vi "Calibrate_Open_All_Freqs-OLD.vi"() -> ()   [LabVIEW 2020]
uses:
  HP 4275A Address constant.vi
panel:
  out "error out":errorcluster
  in  "Cal_Delay_Step":u16
  in  "error in":errorcluster
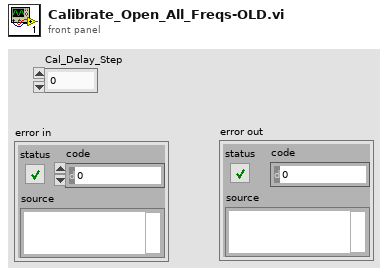
[diagram p1: front panel]
types:
  T1 = typedef "Control 1.ctl" = string
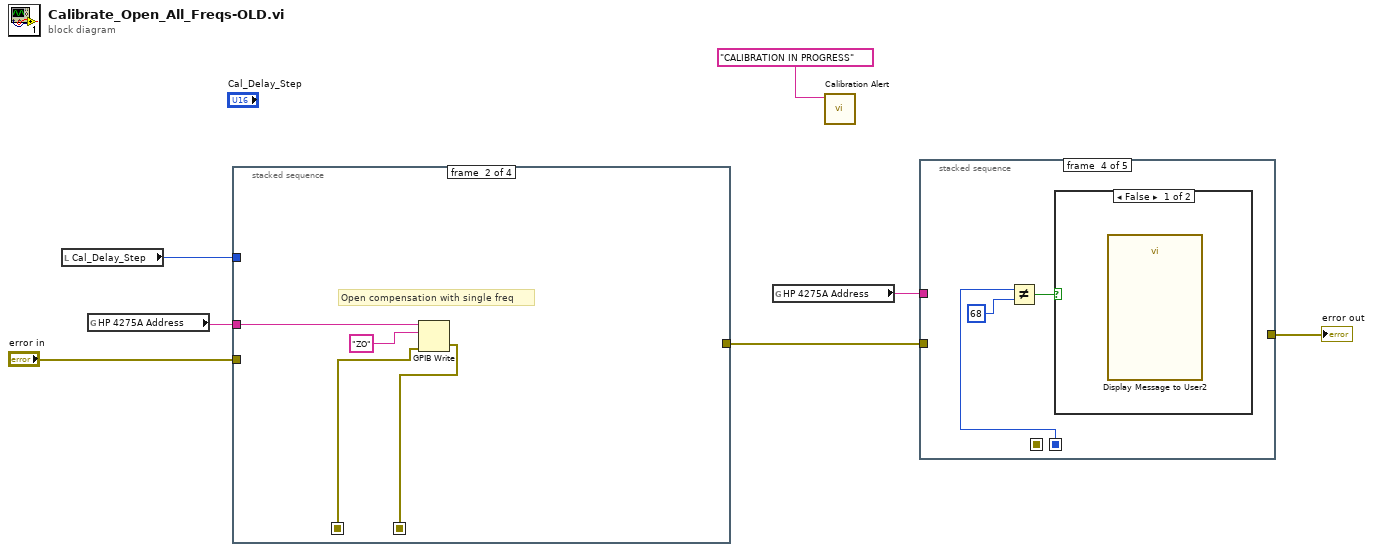
[diagram p0: block diagram]
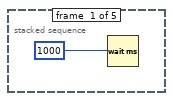
[diagram p2: hidden frame]
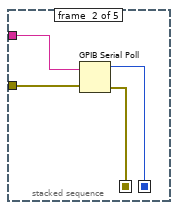
[diagram p3: hidden frame]
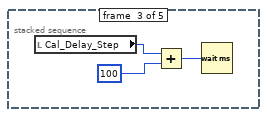
[diagram p4: hidden frame]
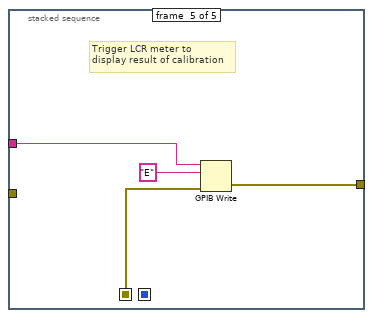
[diagram p6: hidden frame]
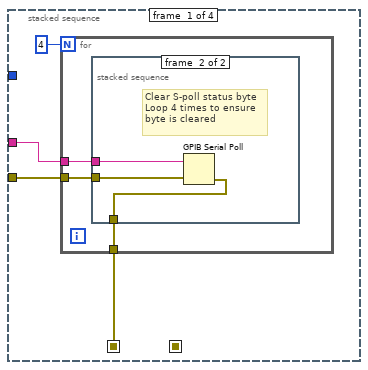
[diagram p7: hidden frame]
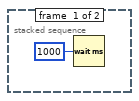
[diagram p8: hidden frame]
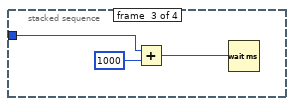
[diagram p9: hidden frame]
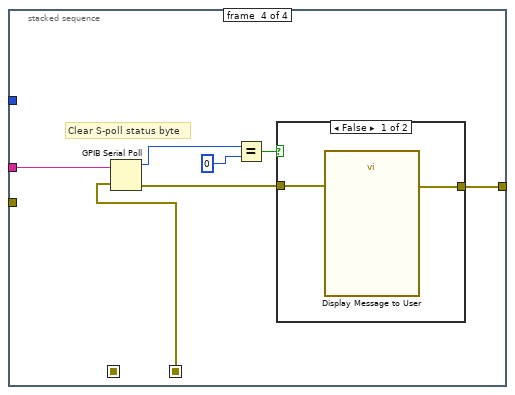
[diagram p10: hidden frame]
diagram:
  n1 = local read "Cal_Delay_Step"() -> (w5:u16)
  n2 = global read "HP 4275A Address constant.vi" "HP 4275A Address"() -> (w7:T1)
  n3 = stacked-sequence {
    seq-local: [w8 _ _ _] -> [_ w20 _ _]
    seq-local: [_ w19 _ _] -> [_ _ _ w31]
    tunnel: w7 -> [w10 w22 _ w32]
    tunnel: "error in" -> [w9 _ _ _]
    tunnel: w5 -> [_ _ w23 _]
    tunnel: [_ _ _ w26] -> w3
    frame #0 {
      n4 = for {
        N: 4 -> [_]
        tunnel: w10 -> [w14]
        tunnel: w9 -> [w13]
        tunnel: [w12] -> w8
        n5 = stacked-sequence {
          tunnel: w14 -> [_ w18]
          tunnel: w13 -> [_ w17]
          tunnel: [_ w16] -> w12
          frame #0 {
            n6 = Wait (ms)(milliseconds to wait=u32 1000) -> ()  [unwired: 1 out]
          }
          frame #1 {
            # "Clear S-poll status byte\nLoop 4 times to ensure\nbyte is cleared"
            n7 = GPIB Serial Poll(0:w18, 1:w17) -> (4:w16:errorcluster)  [unwired: 2 out]
          }
        }
      }
    }
    frame #1 {
      # "Open compensation with single freq"
      n8 = GPIB Write(0:w22, 1:"ZO" ("data"), 3:w20) -> (6:w19:errorcluster)  [unwired: 2 in, 1 out]
    }
    frame #2 {
      n9 = Add(x=w23, y=u16 1000) -> (x+y=w24:u16)
      n10 = Wait (ms)(milliseconds to wait=w24) -> ()  [unwired: 1 out]
    }
    frame #3 {
      # "Clear S-poll status byte"
      n11 = GPIB Serial Poll(0:w32, 1:w31) -> (2:w28:i16, 4:w27:errorcluster)  [unwired: 1 out]
      n12 = Equal?(x=w28, y=i16 0) -> (x = y?=w30:bool)
      n13 = case shown="False" w30 {
        tunnel: w27 -> [w34 w35]
        tunnel: [w33 w35] -> w26
        frame False {
          n14 = call "Display Message to User"("error in (no error)"=w34) -> ("error out"=w33:errorcluster)  [unwired: 9 in, 1 out]
        }
        frame True {
        }
      }
    }
  }
  n15 = global read "HP 4275A Address constant.vi" "HP 4275A Address"() -> (w4:T1)
  n16 = call "Calibration Alert.vi"("message"="CALIBRATION IN PROGRESS" ("format string")) -> ()  [unwired: 10 in, 1 out]
  n17 = stacked-sequence {
    seq-local: [_ w38 _ _ _] -> [_ _ _ w46 _]
    seq-local: [_ w37 _ _ _] -> [_ _ _ _ w48]
    tunnel: w3 -> [_ w39 _ _ _]
    tunnel: w4 -> [_ w40 _ _ w49]
    tunnel: [_ _ _ _ w47] -> w2
    frame #0 {
      n18 = Wait (ms)(milliseconds to wait=u16 1000 ("y")) -> ()  [unwired: 1 out]
    }
    frame #1 {
      n19 = GPIB Serial Poll(0:w40, 1:w39) -> (2:w38:i16, 4:w37:errorcluster)  [unwired: 1 out]
    }
    frame #2 {
      n20 = local read "Cal_Delay_Step"() -> (w43:u16)
      n21 = Add(x=w43, y=u16 100) -> (x+y=w41:u16)
      n22 = Wait (ms)(milliseconds to wait=w41) -> ()  [unwired: 1 out]
    }
    frame #3 {
      n23 = Not Equal?(x=w46, y=i16 68) -> (x != y?=w44:bool)
      n24 = case shown="False" w44 {
        frame False {
          n25 = call "Display Message to User2"() -> ()  [unwired: 10 in, 2 out]
        }
        frame True {
        }
      }
    }
    frame #4 {
      # "Trigger LCR meter to\ndisplay result of calibration"
      n26 = GPIB Write(0:w49, 1:"E" ("data"), 3:w48) -> (6:w47:errorcluster)  [unwired: 2 in, 1 out]
    }
  }
  "error out" <- w2
